vi "Switch_Connect Relay.vi"(8 "error in (no error)":errorcluster, 10 "Connect Pins":string[](array[string])=["K1", "K2", "K7", "K8", "K13", "K14", "K21", "K22", "K23", "K24", "K25", "K26", "K27", "K28"], 11 "Semiconductor Module Context":T1) -> (0 "error out":errorcluster, 3 "Semiconductor Module Context  (dup)":T1)   [LabVIEW 2014]
uses:
  <vilib>/NI_TestStand_SemiconductorModule/NI_TestStand_Semiconductor_Module.lvlibp/PinMap/General/SemiconductorModuleContext.ctl
  <instrlib>/niSwitch/niSwitch.LLB/niSwitch Connect Channels (Single).vi
  <vilib>/NI_TestStand_SemiconductorModule/NI_TestStand_Semiconductor_Module.lvlibp
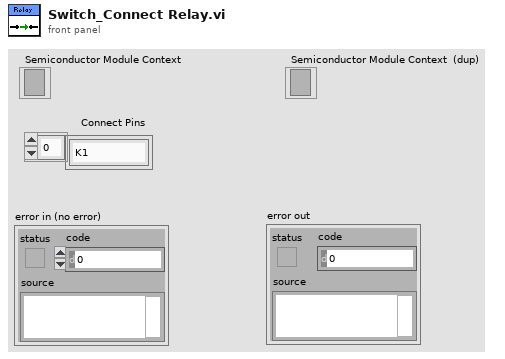
[diagram p1: front panel]
types:
  T1 = typedef "NI_TestStand_Semiconductor_Module.lvlibp/SemiconductorModuleContext.ctl" = refnum<k7>
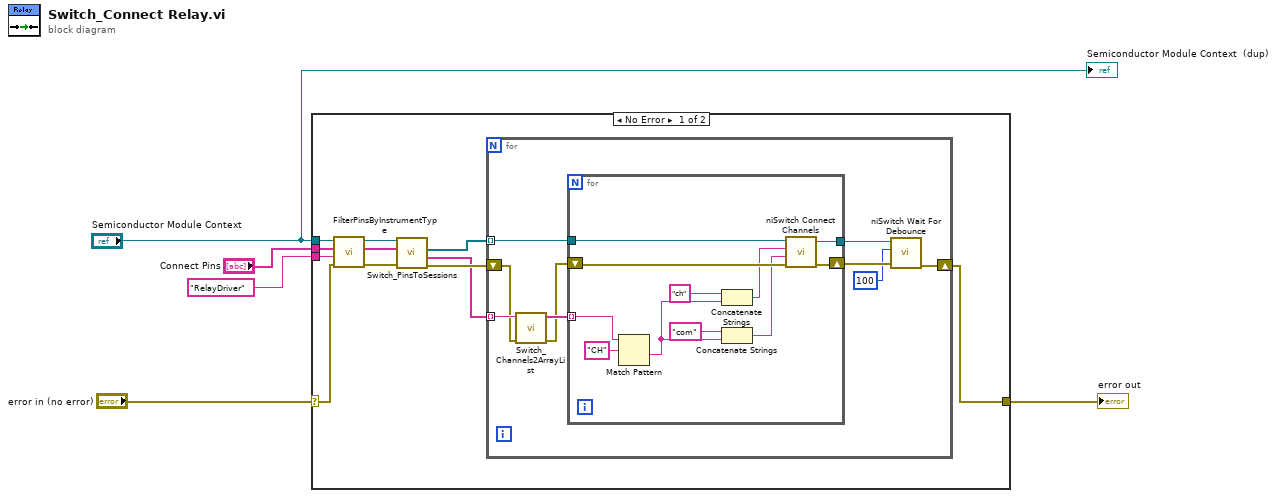
[diagram p0: block diagram]
diagram:
  n1 = case shown="No Error" "error in (no error)" {
    selector: "error in (no error)" -> [w7 w37]
    tunnel: "RelayDriver" -> [w13 _]
    tunnel: "Semiconductor Module Context" -> [w9 _]
    tunnel: "Connect Pins" -> [w8 _]
    tunnel: [w6 w37] -> w2
    frame No Error {
      n2 = call <vilib>:"FilterPinsByInstrumentType.vi"("error in (no error)"=w7, "Instrument Type Id"=w13, "Pins"=w8, "Semiconductor Module Context"=w9) -> ("error out"=w10:errorcluster, "Filtered Pins"=w11:string[], "Semiconductor Module Context Out"=w12:T1)  [unwired: 5 in]
      n3 = call "Switch_PinsToSessions.vi"("error in (no error)"=w10, "Pins"=w11, "Semiconductor Module Context"=w12) -> ("error out"=w16:errorcluster, "Channel Lists"=w15:string[], "Instrument Sessions"=w14:refnum<k15>[])  [unwired: 4 in, 2 out]
      n4 = for {
        shift-right: [w22] -> w6
        shift-left: w16 -> [w18]
        tunnel: w15 -> [w25] mode=indexing
        tunnel: w14 -> [w20] mode=indexing
        n5 = call "Switch_Channels2ArrayList.vi"("error in (no error)"=w18, "Channel List"=w25) -> ("error out"=w17:errorcluster, "Array of Channels"=w24:string[])  [unwired: 8 in]
        n6 = for {
          shift-right: [w31] -> w23
          shift-left: w17 -> [w36]
          tunnel: w24 -> [w27] mode=indexing
          tunnel: [w30] -> w21
          tunnel: w20 -> [w29]
          n7 = Match Pattern(string=w27, regular expression="CH") -> (after substring=w26:string)  [unwired: 1 in, 3 out]
          n8 = Concatenate Strings("ch" ("string"), w26) -> (w33:string)
          n9 = Concatenate Strings("com" ("string"), w26) -> (w32:string)
          n10 = call-poly <instrlib>:"niSwitch Connect Channels.vi"("error in (no error)"=w36, "channel 2"=w32, "channel 1"=w33, "instrument handle"=w29) -> ("error out"=w31:errorcluster, "instrument handle out"=w30:refnum<k15>)  [unwired: 6 in]
        }
        n11 = call <instrlib>:"niSwitch Wait For Debounce.vi"("error in (no error)"=w23, "maximum time (5000 ms)"=100, "instrument handle"=w21) -> ("error out"=w22:errorcluster)  [unwired: 7 in, 1 out]
      }
    }
    frame Error {
    }
  }
  "error out" <- w2
  "Semiconductor Module Context  (dup)" <- "Semiconductor Module Context"
